vi "Lenght (SubVI).vi"(11 "standard error":string) -> (0 "error out":T1)   [LabVIEW 2015]
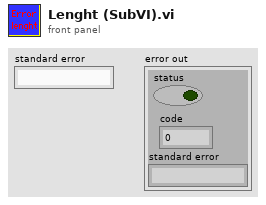
[diagram p1: front panel]
types:
  T1 = cluster{"status":bool, "code":i32, "standard error":string}
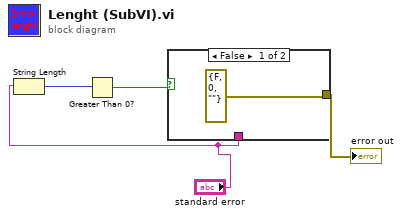
[diagram p0: block diagram]
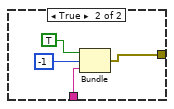
[diagram p2: hidden frame]
diagram:
  n1 = String Length(string="standard error") -> (length=w1:i32)
  n2 = Greater Than 0?(x=w1) -> (x > 0?=w2:bool)
  n3 = case shown="False" w2 {
    tunnel: [errorcluster {"status"=FALSE, "code"=0, "source"=""} ("error constant") w7] -> w3
    tunnel: "standard error" -> [_ w6]
    frame False {
    }
    frame True {
      n4 = Bundle(TRUE, -1, "standard error"=w6) -> (w7:cluster{bool, i32, "standard error":string})  [unwired: 1 in]
    }
  }
  "error out" <- w3
